vi "Init.vi"(8 "error in (no error)":errorcluster, 9 "CtrlRefs":T1, 11 "ExecutionControls in":refnum<class "ExecutionControls.lvclass">) -> (0 "error out":errorcluster, 3 "ExecutionControls out":refnum<class "ExecutionControls.lvclass">)   [LabVIEW 2018, in "ExecutionControls.lvclass"]
uses:
  ExecutionControls.lvclass
  ExecutionCtrlRefs.ctl
  <vilib>/Utility/miscctls.llb/LVForegroundBackgroundColorsTypeDef.ctl
  ExecutionControls.lvclass/ExecutionControls.ctl
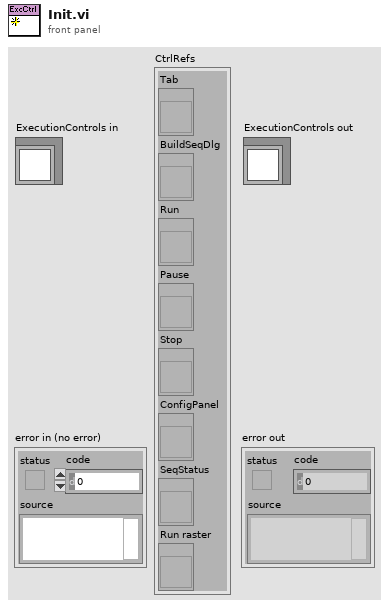
[diagram p1: front panel]
types:
  T1 = typedef "ExecutionCtrlRefs.ctl" = cluster{"Tab":refnum<vi>, "BuildSeqDlg":refnum<vi>, "Run":refnum<vi>, "Pause":refnum<vi>, "Stop":refnum<vi>, "ConfigPanel":refnum<vi>, "SeqStatus":refnum<vi>, "Run raster":refnum<vi>}
  T2 = enum8{"Enabled", "Disabled", "Disabled and Grayed Out"}
  T3 = enum32{"Page Enabled", "Page Disabled", "Page Disabled & Grayed"}
  T4 = enum32{"Sequence Execution", "Manual Control", "Motion Control"}
  T5 = typedef "LVForegroundBackgroundColorsTypeDef.ctl" = cluster{"Foreground Color":u32, "Background Color":u32}
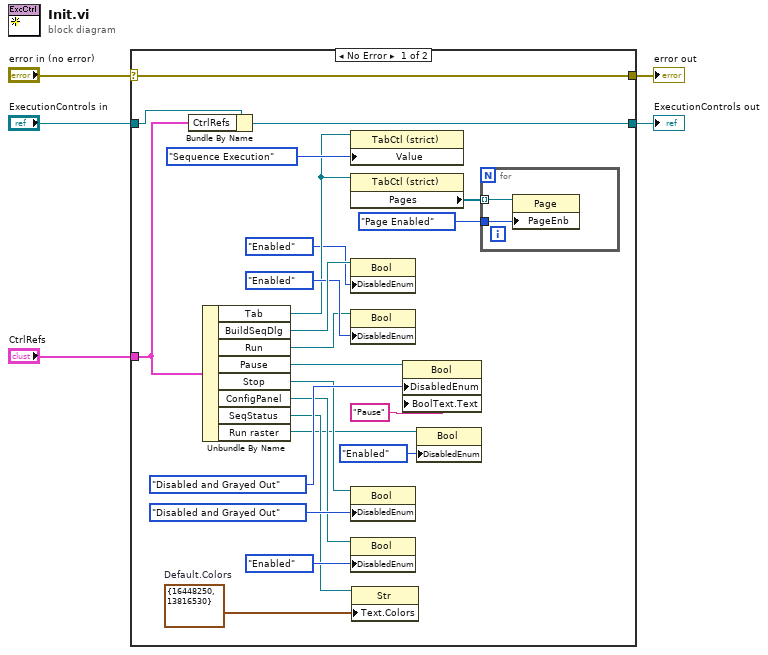
[diagram p0: block diagram]
diagram:
  n1 = case shown="No Error" "error in (no error)" {
    selector: "error in (no error)" -> [w28 w32]
    tunnel: [w28 w32] -> w4
    tunnel: [w26 w31] -> w2
    tunnel: "ExecutionControls in" -> [w27 w31]
    tunnel: "CtrlRefs" -> [w25 _]
    frame No Error {
      w13 = T5 {"Foreground Color"=16448250, "Background Color"=13816530}  # Default.Colors
      n2 = Bundle By Name(cluster=w27, "CtrlRefs"=w25) -> (w26:refnum<class "ExecutionControls.lvclass">)
      n3 = Unbundle By Name(w25) -> ("Tab"=w11:refnum<vi>, "BuildSeqDlg"=w23:refnum<vi>, "Run"=w21:refnum<vi>, "Pause"=w17:refnum<vi>, "Stop"=w16:refnum<vi>, "ConfigPanel"=w15:refnum<vi>, "SeqStatus"=w12:refnum<vi>, "Run raster"=w7:refnum<vi>)
      n4 = property class="TabCtl (strict)"(reference=w11, "Value"=T4."Sequence Execution") -> ()  [unwired: 1 in, 2 out]
      n5 = property class="TabCtl (strict)"(reference=w11) -> ("Pages"=w10:refnum<vi>[])  [unwired: 1 in, 2 out]
      n6 = property class="Bool"(reference=w23, "DisabledEnum"=T2."Enabled" ("Disabled")) -> ()  [unwired: 1 in, 2 out]
      n7 = property class="Bool"(reference=w21, "DisabledEnum"=T2."Enabled" ("Disabled")) -> ()  [unwired: 1 in, 2 out]
      n8 = property class="Bool"(reference=w16, "DisabledEnum"=T2."Disabled and Grayed Out" ("Disabled")) -> ()  [unwired: 1 in, 2 out]
      n9 = property class="Bool"(reference=w15, "DisabledEnum"=T2."Enabled" ("Disabled")) -> ()  [unwired: 1 in, 2 out]
      n10 = property class="Str"(reference=w12, "Text.Colors"=w13) -> ()  [unwired: 1 in, 2 out]
      n11 = property class="Bool"(reference=w17, "DisabledEnum"=T2."Disabled and Grayed Out" ("Disabled"), "BoolText.Text"="Pause" ("Boolean Text.Text")) -> ()  [unwired: 1 in, 2 out]
      n12 = property class="Bool"(reference=w7, "DisabledEnum"=T2."Enabled" ("Disabled")) -> ()  [unwired: 1 in, 2 out]
      n13 = for {
        tunnel: w10 -> [w30] mode=indexing
        tunnel: T3."Page Enabled" ("Page Enabled State") -> [w29]
        n14 = property class="Page"(reference=w30, "PageEnb"=w29) -> ()  [unwired: 1 in, 2 out]
      }
    }
    frame Error {
    }
  }
  "error out" <- w4
  "ExecutionControls out" <- w2
